vi "Verify image path.vi"(8 "error in (no error)":errorcluster, 11 "Channel in":refnum<class "Channel.lvclass">) -> (0 "error out":errorcluster, 3 "Channel out":refnum<class "Channel.lvclass">)   [LabVIEW 2018, in "Channel.lvclass"]
uses:
  Channel.lvclass
  Channel.lvclass/Channel.ctl
  Simulated_CCD_Camera/Simulated_CCD_Camera.lvclass/Simulated_CCD_Camera.ctl
  <vilib>/ErrorRing/Error Ring.xnode
  Simulated_CCD_Camera/Simulated_CCD_Camera.lvclass
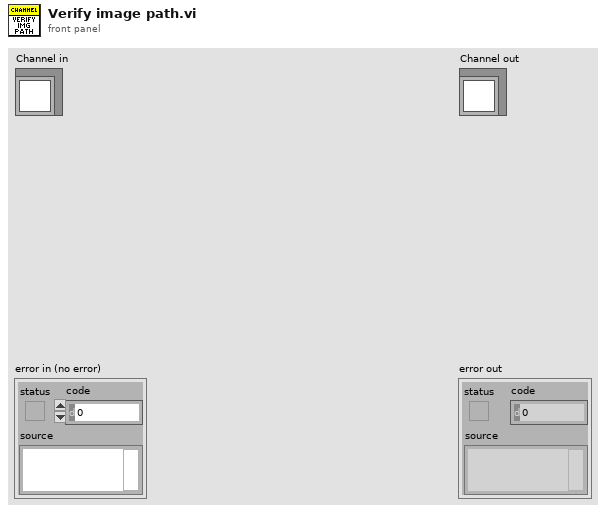
[diagram p1: front panel]
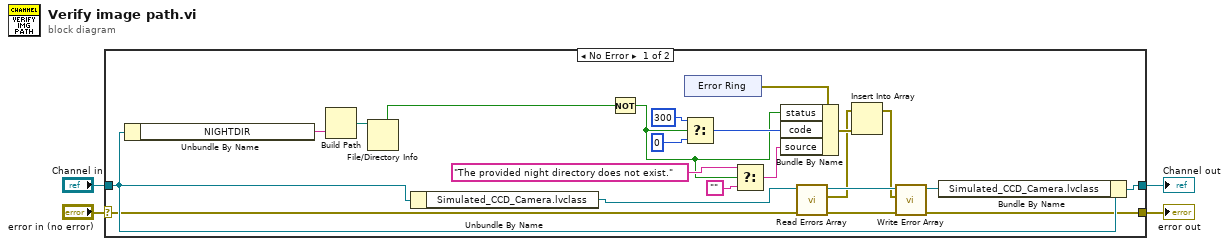
[diagram p0: block diagram]
diagram:
  n1 = case shown="No Error" "error in (no error)" {
    selector: "error in (no error)" -> [w22 w29]
    tunnel: [w9 w29] -> w3
    tunnel: [w23 w28] -> w1
    tunnel: "Channel in" -> [w24 w28]
    frame No Error {
      n2 = Unbundle By Name(w24) -> ("NIGHTDIR"=w26:string)
      n3 = Build Path(name or relative path=w26) -> (appended path=w25:path)  [unwired: 1 in]
      n4 = File/Directory Info(path=w25) -> (directory=w17:bool)  [unwired: 1 in, 6 out]
      n5 = Unbundle By Name(w24) -> ("Simulated_CCD_Camera.lvclass"=w18:refnum<class "Simulated_CCD_Camera.lvclass">)
      n6 = Not(x=w17) -> (.not. x?=w11:bool)
      n7 = xnode "Error Ring"() -> ("error out"=w5:errorcluster)
      n8 = Select(t=300 ("code"), s=w11, f=0 ("code")) -> (s? t:f=w15:i32)
      n9 = Select(t="The provided night directory does not exist." ("source"), s=w11, f="") -> (s? t:f=w10:string)
      n10 = Bundle By Name(cluster=w5, "status"=w11, "code"=w15, "source"=w10) -> (w8:errorcluster)
      n11 = call "Read Errors Array.vi"("error in (no error)"=w22, "Simulated_CCD_Camera in"=w18) -> ("error out"=w20:errorcluster, "Errors array"=w7:errorcluster[], "Simulated_CCD_Camera out"=w21:refnum<class "Simulated_CCD_Camera.lvclass">)  [unwired: 7 in]
      n12 = Insert Into Array(array=w7, new element=w8) -> (w6:errorcluster[])  [unwired: 1 in]
      n13 = call "Write Error Array.vi"("error in (no error)"=w20, "Errors array"=w6, "Simulated_CCD_Camera in"=w21) -> ("error out"=w9:errorcluster, "Simulated_CCD_Camera out"=w19:refnum<class "Simulated_CCD_Camera.lvclass">)  [unwired: 7 in]
      n14 = Bundle By Name(cluster=w24, "Simulated_CCD_Camera.lvclass"=w19) -> (w23:refnum<class "Channel.lvclass">)
    }
    frame Error {
    }
  }
  "error out" <- w3
  "Channel out" <- w1
